vi "TaskBarMode.vi"() -> ()   [LabVIEW 2020]
uses:
  C:/Users/dzoni/Documents/NJ/Playground/LV/WinAPI/DLL/WinAPI.dll
  DLL/WinAPI.dll
panel:
  out "GetTaskbarState":i32(ring)=1 items=["AutoHide"=1, "AlwaysOnTop"=2]
  in  "option":i32(ring)=2 items=["AutoHide"=1, "AlwaysOnTop"=2]
  out "GetTaskbarState 2":i32(ring)=1 items=["AutoHide"=1, "AlwaysOnTop"=2]
  out "error out":errorcluster
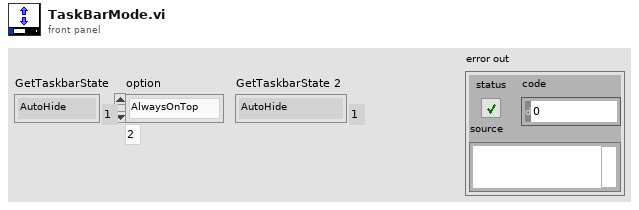
[diagram p1: front panel]
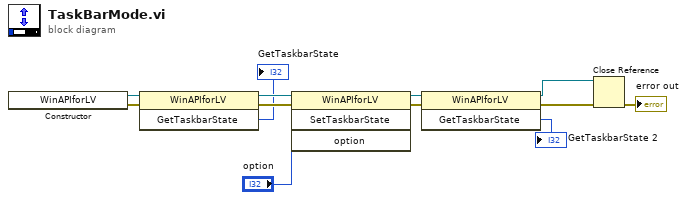
[diagram p0: block diagram]
diagram:
  n1 = constructor class="WinAPIforLV"() -> (reference out=w10:refnum<k24>, error out=w9:errorcluster)  [unwired: 3 in, 1 out]
  n2 = invoke class="WinAPIforLV" method="GetTaskbarState"(reference=w10, error in=w9) -> (reference out=w3:refnum<k24>, error out=w2:errorcluster, "GetTaskbarState"=→"GetTaskbarState":i32)  [unwired: 1 in]
  n3 = invoke class="WinAPIforLV" method="SetTaskbarState"(reference=w3, error in=w2, "option"="option") -> (reference out=w8:refnum<k24>, error out=w7:errorcluster)  [unwired: 1 in, 2 out]
  n4 = invoke class="WinAPIforLV" method="GetTaskbarState"(reference=w8, error in=w7) -> (reference out=w6:refnum<k24>, error out=w5:errorcluster, "GetTaskbarState"=→"GetTaskbarState 2":i32)  [unwired: 1 in]
  n5 = Close Reference(reference=w6, error in (no error)=w5) -> (error out=→"error out":errorcluster)
